vi "Pulse Acquired Response.vi"(8 "error in (no error)":errorcluster, 9 "Acquired":bool, 10 "Sender":string, 11 "Pulse Controller in":refnum<class "Pulse Controller.lvclass">) -> (0 "error out":errorcluster, 3 "Pulse Controller out":refnum<class "Pulse Controller.lvclass">)   [LabVIEW 2021, in "Pulse Controller.lvclass"]
uses:
  Pulse Controller.lvclass
  C:/GitHub/LabActor/Controllers/Process Controller/Process Controller.lvclass
  Process Controller/Process Controller.lvclass/Process Controller.ctl
  Pulse Controller.lvclass/Pulse Controller.ctl
  Process Controller/Request type.ctl
  Process Controller/Read Active measurements names.vi
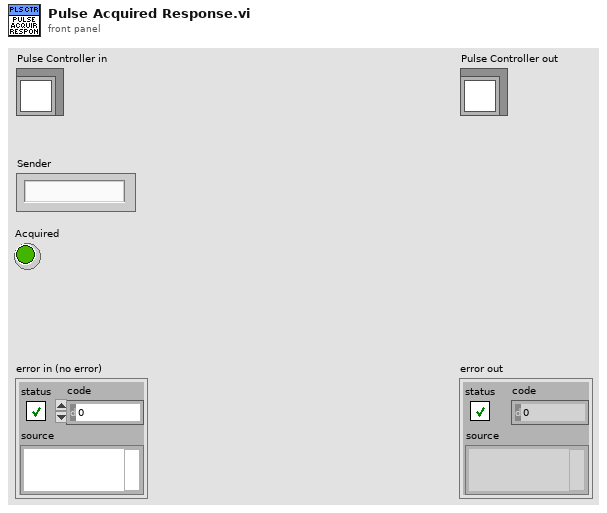
[diagram p1: front panel]
types:
  T1 = typedef "Request type.ctl" = enum16{"Process complete", "User command", "Auto-restart", "Error"}
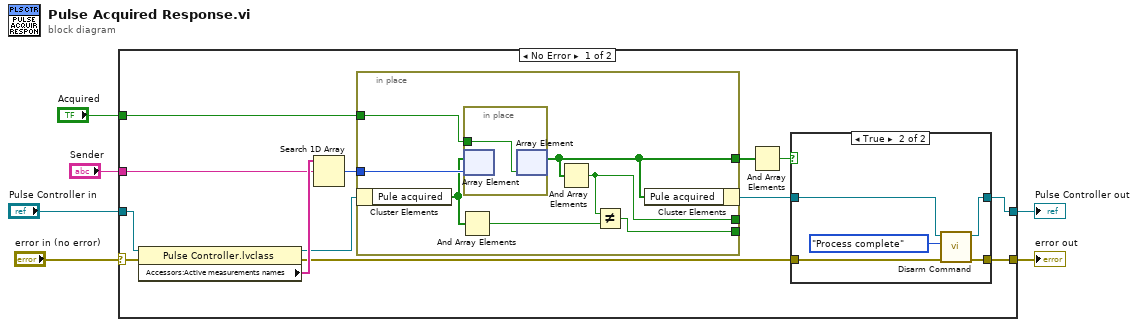
[diagram p0: block diagram]
diagram:
  n1 = case shown="No Error" "error in (no error)" {
    selector: "error in (no error)" -> [w8 w36]
    tunnel: [w7 w36] -> w5
    tunnel: [w10 w35] -> w3
    tunnel: "Pulse Controller in" -> [w14 w35]
    tunnel: "Acquired" -> [w16 _]
    tunnel: "Sender" -> [w15 _]
    frame No Error {
      n2 = property class="Pulse Controller.lvclass"(reference=w14, error in=w8) -> (reference out=w17:refnum<class "Pulse Controller.lvclass">, error out=w9:errorcluster, "Accessors:Active measurements names"=w19:string[])
      n3 = Search 1D Array(1D array=w19, element=w15) -> (index of element=w18:i32)  [unwired: 1 in]
      n4 = in-place {
        in-place-border: w18 -> [w33]
        in-place-border: w16 -> [w32]
        in-place-border: [w29] -> _
        in-place-border: [w28] -> _
        in-place-border: [w27] -> w13
        n5 = in-place-cluster #1(w17) -> ("Pule acquired"=w31:bool[])
        n6 = And Array Elements(Boolean array=w31) -> (logical AND=w30:bool)
        n7 = in-place {
          in-place-border: w32 -> [w34]
          n8 = in-place-array #2(w31, w33) -> ()  [unwired: 1 out]
          n9 = in-place-array #2(w34) -> (w27:bool[])  [unwired: 1 out]
        }
        n10 = And Array Elements(Boolean array=w27) -> (logical AND=w28:bool)
        n11 = Not Equal?(x=w28, y=w30) -> (x != y?=w29:bool)
        n12 = in-place-cluster #1("Pule acquired"=w27) -> (w11:refnum<class "Pulse Controller.lvclass">)
      }
      n13 = And Array Elements(Boolean array=w13) -> (logical AND=w12:bool)
      n14 = case shown="True" w12 {
        tunnel: w11 -> [w21 w26]
        tunnel: [w21 w25] -> w10
        tunnel: w9 -> [w20 w24]
        tunnel: [w20 w23] -> w7
        frame False {
        }
        frame True {
          n15 = call-dynamic "Disarm Command.vi"("error in (no error)"=w24, "Request type"=Request_type."Process complete", "Pulse Controller in"=w26) -> ("error out"=w23:errorcluster, "Pulse Controller out"=w25:refnum<class "Pulse Controller.lvclass">)  [unwired: 7 in]
        }
      }
    }
    frame Error {
    }
  }
  "error out" <- w5
  "Pulse Controller out" <- w3
